vi "R45_2-RT.vi"() -> ()   [LabVIEW 2016]
uses:
  <vilib>/rvi/interface/nirviOpenFPGA/nirviOpenFPGA.xnode
  <vilib>/rvi/interface/nirviReadWriteControl/nirviReadWriteControl.xnode
  R45_2-FPGA.vi
  Controls/GP307 cluster.ctl
  <vilib>/functionblocks/FB Core/FB Core.xnode
  <vilib>/functionblocks/Control/PID/PID.vi
  <vilib>/functionblocks/NI_FunctionBlock Libraries.lvlib
  Controls/Glassman Control.ctl
  NiFpgaLv.dll
  <vilib>/Utility/error.llb/Error Cluster From Error Code.vi
  <vilib>/rvi/errors/niLvFpgaAdjustHostInterfaceError.vi
  Controls/GV states.ctl
  Controls/Aperture states.ctl
  Controls/Faraday cup states.ctl
  <vilib>/NI_Real-Time Target Support.lvlib
  FPGA Bitfiles/PRIMEControl2017_FPGATarget8_R45-2-FPGA_U4jwOoavuXQ.lvbitx
  <vilib>/FPGAPlugInAG/cRIO-9074/niLvFpga_Open_cRIO-9074.vi
panel:
  in  "Tab Control":T1(tab)
  out "R45 ExB 1 HV Enable":bool
  out "R45 ExB 1 voltage set":dbl
  out "ExB 1- I read":dbl
  out "ExB 1- V read":dbl
  out "ExB 2+ I read":dbl
  out "ExB 2+ V read":dbl
  out "ExB 2- I read":dbl
  out "ExB 2- V read":dbl
  out "R45 ExB 2 HV Enable":bool
  out "R45 ExB 2 voltage set":dbl
  out "X-Steerer Magnet current set":dbl
  out "ExB 1+ I read":dbl
  out "ExB 1+ V read":dbl
  out "GRM magnet current set":dbl
  out "GFM read string":string
  in  "proportional gain (Kc) - GFM":dbl=1.0
  in  "integral time (Ti, min) - GFM":dbl=0.01
  in  "derivative time (Td, min) - GFM":dbl
  in  "output high - GFM":dbl=205.0
  in  "output low - GFM":dbl
  out "GFM field read":u8[](array[numeric])
  out "GFM field":dbl format="%#_8f"
  out "GFM command":u8[](array[numeric])
  out "R45 ExB 2 command string":string
  out "R45 ExB 2 command array":u8[](array[numeric])
  out "ExB #2 magnet current set":dbl
  out "GFM command string":string
  out "GFM field set":dbl
  out "ExB #1 magnet current set":dbl
  out "R45 ExB 1 command string":string
  out "R45 ExB 1 command array":u8[](array[numeric])
  out "X-steerer Mag V read":dbl
  out "X-steerer Mag I read":dbl
  out "Ion Gauge 3-2":u8[](array[numeric])
  out "Convectron gauge 3-2":u8[](array[numeric])
  out "Ion gauge 2-2":u8[](array[numeric])
  out "Ion gauge 2-1":u8[](array[numeric])
  out "Convectron 3-1":u8[](array[numeric])
  out "Ion gauge 3-1":u8[](array[numeric])
  out "Convectron 2-2":u8[](array[numeric])
  out "Convectron 2-1":u8[](array[numeric])
  out "Ion Gauge 4-1":u8[](array[numeric])
  out "Convectron Gauge 4-1":u8[](array[numeric])
  out "Ion Gauge 4-2":u8[](array[numeric])
  out "Convectron Gauge 4-2":u8[](array[numeric])
  out "R45 Quad  vac gauge cluster":T2
  out "R45 Detector vac gauge cluster":T2
  out "R45 ExB Slot vac gauge cluster":T2
  out "Vac cluster 2 Ion Guage Interlock":bool
  out "Vac cluster 3 Ion Guage Interlock":bool
  out "Vac cluster 4 Ion Guage Interlock":bool
  out "Vac cluster 1 Gauge Interlock":bool
  out "Vac cluster 1 Interlock bypass":bool
  out "Switch Object Vac Interlock":bool
  out "Switch Object Interlock Bypass":bool
  out "Vac cluster 2 Interlock bypass":bool
  out "Vac cluster 4 Interlock bypass":bool
  out "Vac cluster 3 Interlock bypass":bool
  out "Turbo 2 GV Status":T3
  out "Turbo 1 GV Status":T3
  out "Beamline GV 3 Status":T3
  out "Beamline GV 2 Status":T3
  out "R45 Switching Mag GV Status":T3
  out "Turbo 3 GV Status":T3
  out "Detector FC status":T4
  out "Detector Aperture status":T5
  out "Detector Aperture Position":cluster{"IN sensor":bool, "OUT sensor":bool}
  out "Turbo 3 GV Status":T6
  out "Turbo 2 GV Status":T6
  out "Beamline GV 3 Status":T6
  out "Turbo 1 GV Status":T6
  out "R45 Switching Mag GV Status":T6
  out "ExB Slot Aperture Position":cluster{"IN sensor":bool, "OUT sensor":bool}
  out "Detector FC Position":cluster{"IN sensor":bool, "OUT sensor":bool}
  out "Beamline GV 2 Status":T6
  out "ExB Slot Aperture Status":T5
  out "R45 Detector FC insert":bool
  out "R45 Detector Aperture insert":bool
  out "R45 ExB Slot Aperture insert":bool
  out "R45 Turbo 3 GV":bool
  out "R45 Turbo 2 GV":bool
  out "R45 Switching Magnet GV":bool
  out "R45 Turbo 1 GV":bool
  out "R45 Beamline GV 3":bool
  out "R45 Beamline GV 2":bool
  out "HV control loop error":errorcluster
  out "HV readback loop error":errorcluster
  out "Error Reporter":errorcluster
  out "ExB 1 PS loop error":errorcluster
  out "ExB 2 PS loop error":errorcluster
  out "GFM loop error":errorcluster
  out "Interlock readbacks Loop error":errorcluster
  out "Vacuum readback error":errorcluster
  out "Actuator loop error":errorcluster
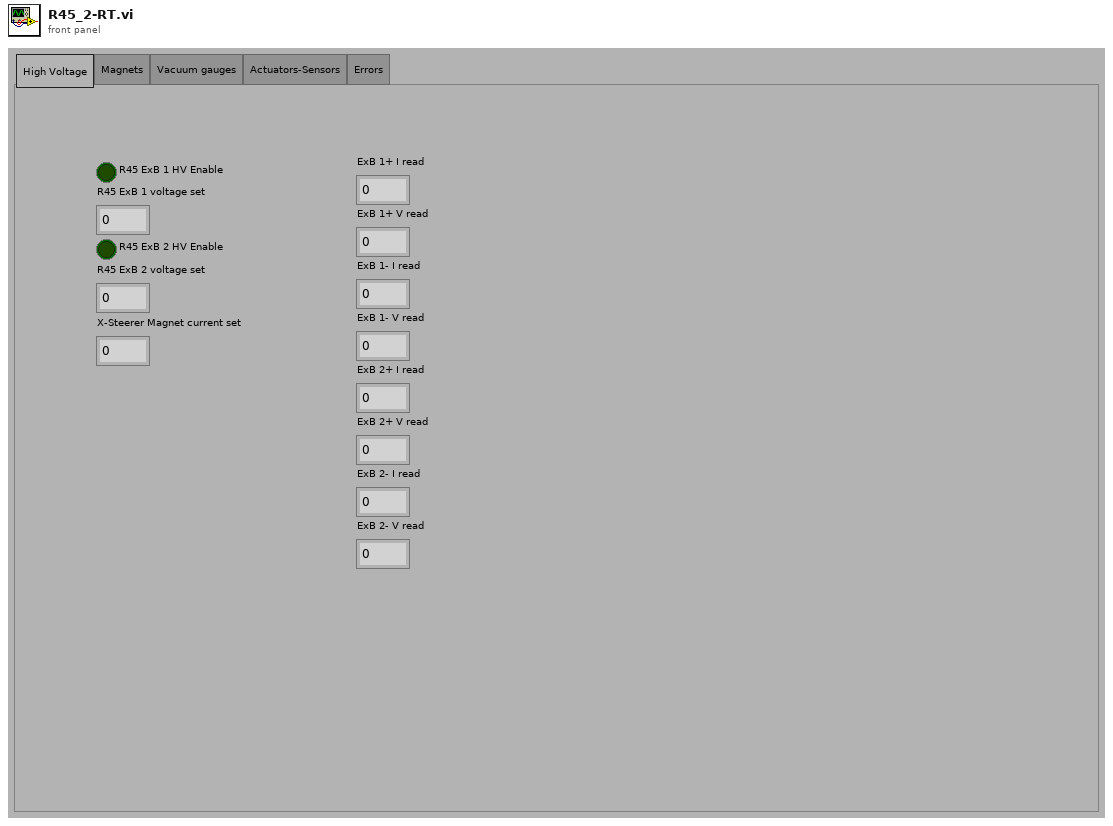
[diagram p1: front panel]
types:
  T1 = enum32{"High Voltage", "Magnets", "Vacuum gauges", "Actuators-Sensors", "Errors"}
  T2 = cluster{"Ion gauge 1":string, "Convectron  Gauge 1 ":string, "Ion Gauge 2":string, "Convectrom Gauge 2":string}
  T3 = typedef "GV states.ctl" = enum16{"status unclear", "closed", "open"}
  T4 = typedef "Faraday cup states.ctl" = enum16{"FC status unclear", "FC in", "FC out"}
  T5 = typedef "Aperture states.ctl" = enum16{"Aperture status unclear", "Aperture in", "Aperture out"}
  T6 = cluster{"OPEN sensor":bool, "Closed sensor":bool}
  T7 = typedef "Glassman Control.ctl" = cluster{"V-program":fxp<+/-,16,5>, "HV Enable":bool}
  T8 = cluster{"I-monitor":fxp<+/-,16,5>, "V-monitor":fxp<+/-,16,5>}
  T9 = typedef "GP307 cluster.ctl" = cluster{"Ion gauge 1":string, "Convectron  Gauge 1 ":string, "Ion Gauge 2":string, "Convectrom Gauge 2":string}
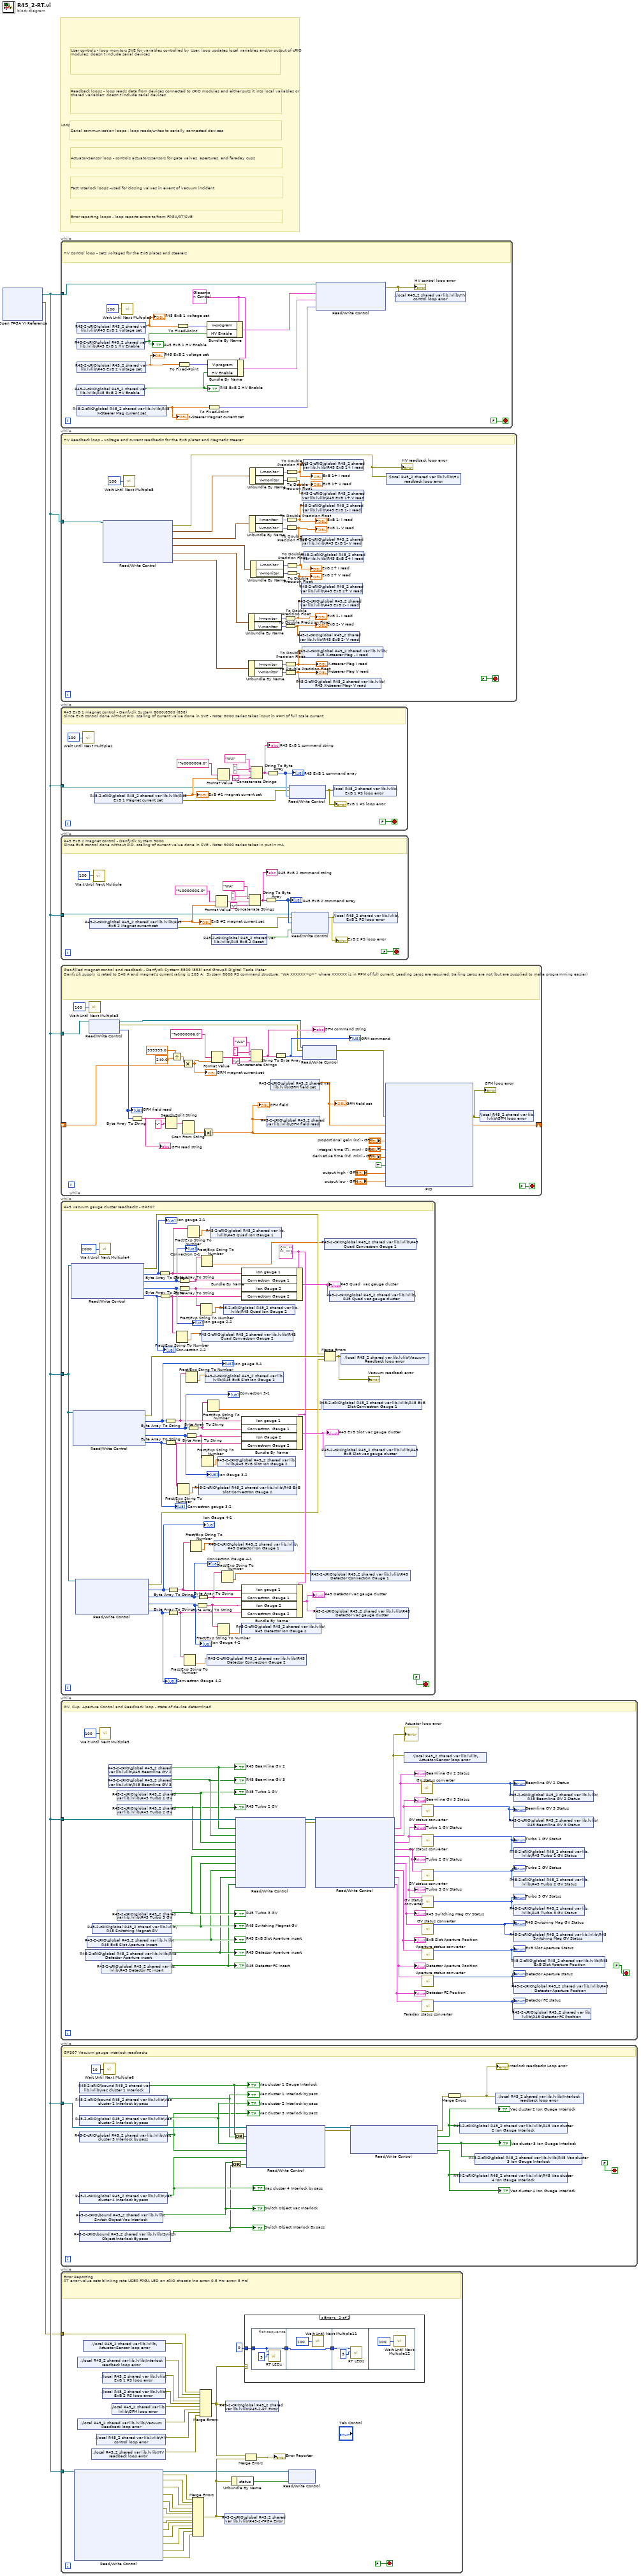
[diagram p0: block diagram]
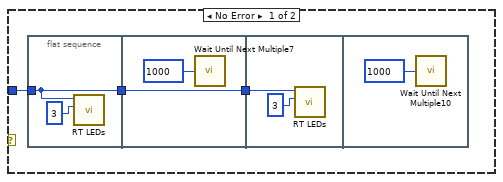
[diagram p2: hidden frame]
diagram:
  # "Serial communication loops - loop reads/writes to serially connected devices"
  # "Actuator-Sensor loop - controls actuators/sensors for gate valves, apertures, and faraday cups"
  # "Fast Interlock loops -used for closing valves in event of vacuum incident"
  # "Error reporting loops - loop reports errors to/from FPGA/RT/SVE"
  # "Readback loops - loop reads data from devices connected to cRIO modules and either puts it into local variables or shared variables; doesn't include serial devices"
  # "User controls - loop monitors SVE for variables controlled by User; loop updates local variables and/or output of cRIO modules; doesn't include serial devices"
  # "Loop legend - loops are color coded by responsibility"
  n1 = xnode "Open FPGA VI Reference"() -> ("FPGA VI Reference Out"=w2:refnum<k20>, "error out"=w1:errorcluster)  [unwired: 2 in]
  n2 = while {
    tunnel: w2 -> [w17]
    stop <- FALSE stop-if-true
    w13 = T7 {"V-program"=0.0, "HV Enable"=FALSE} ("Glassman Control")
    # "HV Control loop - sets voltages for the ExB plates and steerers"
    n3 = shared-variable "R45-2-cRIO\\global R45_2 shared var lib.lvlib\\R45 ExB 1 voltage set"() -> (w10:dbl)  [unwired: 1 in, 1 out]
    "R45 ExB 1 voltage set" <- w10
    n4 = shared-variable "R45-2-cRIO\\global R45_2 shared var lib.lvlib\\R45 ExB 1 HV Enable"() -> (w11:bool)  [unwired: 1 in, 1 out]
    "R45 ExB 1 HV Enable" <- w11
    n5 = shared-variable "R45-2-cRIO\\global R45_2 shared var lib.lvlib\\R45 ExB 2 voltage set"() -> (w8:dbl)  [unwired: 1 in, 1 out]
    "R45 ExB 2 voltage set" <- w8
    n6 = shared-variable "R45-2-cRIO\\global R45_2 shared var lib.lvlib\\R45 ExB 2 HV Enable"() -> (w6:bool)  [unwired: 1 in, 1 out]
    "R45 ExB 2 HV Enable" <- w6
    n7 = shared-variable "R45-2-cRIO\\global R45_2 shared var lib.lvlib\\R45 X-Steerer Mag current set"() -> (w16:dbl)  [unwired: 1 in, 1 out]
    "X-Steerer Magnet current set" <- w16
    n8 = call "Wait Until Next Multiple9"("Count(mSec)"=u32 100 ("millisecond multiple")) -> ()  [unwired: 1 out]
    n9 = To Fixed-Point(number=w10) -> (fixed-point=w9:fxp<+/-,20,5>)  [unwired: 1 in]
    n10 = To Fixed-Point(number=w8) -> (fixed-point=w7:fxp<+/-,20,5>)  [unwired: 1 in]
    n11 = Bundle By Name(cluster=w13, "V-program"=w9, "HV Enable"=w11) -> (w12:T7)
    n12 = Bundle By Name(cluster=w13, "V-program"=w7, "HV Enable"=w6) -> (w14:T7)
    n13 = To Fixed-Point(number=w16) -> (fixed-point=w15:fxp<+/-,20,5>)  [unwired: 1 in]
    n14 = xnode "Read/Write Control"("FPGA VI Reference In"=w17, "ExB 1 - Voltage Set"=w12, "ExB 2 - Voltage Set"=w14, "Mag Steerer I-program"=w15) -> ("error out"=w5:errorcluster)  [unwired: 1 in, 1 out]
    "HV control loop error" <- w5
    n15 = shared-variable ".\\local R45_2 shared var lib.lvlib\\HV control loop error"(w5) -> ()  [unwired: 1 in, 1 out]
  }
  n16 = while {
    tunnel: w2 -> [w46]
    stop <- FALSE stop-if-true
    # "HV Readback loop - voltage and current readbacks for the ExB plates and Magnetic steerer"
    n17 = xnode "Read/Write Control"("FPGA VI Reference In"=w46) -> ("error out"=w28:errorcluster, "ExB 1+ Monitor"=w45:T8, "ExB 1- Monitor"=w44:T8, "ExB 2+ Monitor"=w43:T8, "ExB 2- Monitor"=w42:T8, "Mag Steerer - Monitor"=w41:T8)  [unwired: 1 in, 1 out]
    "HV readback loop error" <- w28
    n18 = call "Wait Until Next Multiple8"("Count(mSec)"=u32 100 ("millisecond multiple")) -> ()  [unwired: 1 out]
    n19 = Unbundle By Name(w42) -> ("I-monitor"=w35:fxp<+/-,16,5>, "V-monitor"=w34:fxp<+/-,16,5>)
    n20 = Unbundle By Name(w41) -> ("I-monitor"=w33:fxp<+/-,16,5>, "V-monitor"=w32:fxp<+/-,16,5>)
    n21 = Unbundle By Name(w44) -> ("I-monitor"=w39:fxp<+/-,16,5>, "V-monitor"=w38:fxp<+/-,16,5>)
    n22 = Unbundle By Name(w45) -> ("I-monitor"=w31:fxp<+/-,16,5>, "V-monitor"=w40:fxp<+/-,16,5>)
    n23 = Unbundle By Name(w43) -> ("I-monitor"=w37:fxp<+/-,16,5>, "V-monitor"=w36:fxp<+/-,16,5>)
    n24 = To Double Precision Float(number=w35) -> (double precision float=w22:dbl)
    "ExB 2- I read" <- w22
    n25 = To Double Precision Float(number=w34) -> (double precision float=w21:dbl)
    "ExB 2- V read" <- w21
    n26 = To Double Precision Float(number=w33) -> (double precision float=w20:dbl)
    "X-steerer Mag I read" <- w20
    n27 = To Double Precision Float(number=w32) -> (double precision float=w19:dbl)
    "X-steerer Mag V read" <- w19
    n28 = To Double Precision Float(number=w39) -> (double precision float=w26:dbl)
    "ExB 1- I read" <- w26
    n29 = To Double Precision Float(number=w38) -> (double precision float=w25:dbl)
    "ExB 1- V read" <- w25
    n30 = To Double Precision Float(number=w31) -> (double precision float=w29:dbl)
    "ExB 1+ I read" <- w29
    n31 = To Double Precision Float(number=w40) -> (double precision float=w30:dbl)
    "ExB 1+ V read" <- w30
    n32 = To Double Precision Float(number=w37) -> (double precision float=w24:dbl)
    "ExB 2+ I read" <- w24
    n33 = To Double Precision Float(number=w36) -> (double precision float=w23:dbl)
    "ExB 2+ V read" <- w23
    n34 = shared-variable "R45-2-cRIO\\global R45_2 shared var lib.lvlib\\R45 ExB 2- V read"(w21) -> ()  [unwired: 1 in, 1 out]
    n35 = shared-variable "R45-2-cRIO\\global R45_2 shared var lib.lvlib\\R45 X-steerer Mag- V read"(w19) -> ()  [unwired: 1 in, 1 out]
    n36 = shared-variable "R45-2-cRIO\\global R45_2 shared var lib.lvlib\\R45 ExB 2+ V read"(w23) -> ()  [unwired: 1 in, 1 out]
    n37 = shared-variable "R45-2-cRIO\\global R45_2 shared var lib.lvlib\\R45 ExB 2- I read"(w22) -> ()  [unwired: 1 in, 1 out]
    n38 = shared-variable "R45-2-cRIO\\global R45_2 shared var lib.lvlib\\R45 ExB 1- V read"(w25) -> ()  [unwired: 1 in, 1 out]
    n39 = shared-variable "R45-2-cRIO\\global R45_2 shared var lib.lvlib\\R45 X-steerer Mag - I read"(w20) -> ()  [unwired: 1 in, 1 out]
    n40 = shared-variable "R45-2-cRIO\\global R45_2 shared var lib.lvlib\\R45 ExB 1+ V read"(w30) -> ()  [unwired: 1 in, 1 out]
    n41 = shared-variable "R45-2-cRIO\\global R45_2 shared var lib.lvlib\\R45 ExB 1- I read"(w26) -> ()  [unwired: 1 in, 1 out]
    n42 = shared-variable "R45-2-cRIO\\global R45_2 shared var lib.lvlib\\R45 ExB 1+ I read"(w29) -> ()  [unwired: 1 in, 1 out]
    n43 = shared-variable "R45-2-cRIO\\global R45_2 shared var lib.lvlib\\R45 ExB 2+ I read"(w24) -> ()  [unwired: 1 in, 1 out]
    n44 = shared-variable ".\\local R45_2 shared var lib.lvlib\\HV readback loop error"(w28) -> ()  [unwired: 1 in, 1 out]
  }
  n45 = while {
    tunnel: w2 -> [w50]
    stop <- FALSE stop-if-true
    # "R45 ExB 1 magnet control - Danfysik System 8000/8500 (858)\nSince ExB control done without PID, scaling of current value done in SVE - Note: 8000 series takes input in PPM of full scale current"
    n46 = call "Wait Until Next Multiple2"("Count(mSec)"=u32 100 ("millisecond multiple")) -> ()  [unwired: 1 out]
    n47 = shared-variable "R45-2-cRIO\\global R45_2 shared var lib.lvlib\\R45 ExB 1 Magnet current set"() -> (w57:dbl, error out=w51:errorcluster)  [unwired: 1 in]
    "ExB #1 magnet current set" <- w57
    n48 = Format Value(format string="%0000006.0", value (0)=w57) -> (output string=w55:string)  [unwired: 1 out]
    n49 = Concatenate Strings("WA", " ", w55, "\r") -> (w58:string)
    "R45 ExB 1 command string" <- w58
    n50 = String To Byte Array(string=w58) -> (unsigned byte array=w56:u8[])
    "R45 ExB 1 command array" <- w56
    n51 = xnode "Read/Write Control"("FPGA VI Reference In"=w50, "error in"=w51, "ExB 1 PS set"=w56) -> ("error out"=w48:errorcluster)  [unwired: 1 out]
    "ExB 1 PS loop error" <- w48
    n52 = shared-variable ".\\local R45_2 shared var lib.lvlib\\ExB 1 PS loop error"(w48) -> ()  [unwired: 1 in, 1 out]
  }
  n53 = while {
    tunnel: w2 -> [w62]
    stop <- FALSE stop-if-true
    # "R45 ExB 2 magnet control - Danfysik System 9000\nSince ExB control done without PID, scaling of current value done in SVE - Note: 9000 series takes in put in mA"
    n54 = shared-variable "R45-2-cRIO\\global R45_2 shared var lib.lvlib\\R45 ExB 2 Magnet current set"() -> (w70:dbl, error out=w64:errorcluster)  [unwired: 1 in]
    "ExB #2 magnet current set" <- w70
    n55 = call "Wait Until Next Multiple"("Count(mSec)"=u32 100 ("millisecond multiple")) -> ()  [unwired: 1 out]
    n56 = shared-variable "R45-2-cRIO\\global R45_2 shared var lib.lvlib\\R45 ExB 2 Reset"() -> (w73:bool)  [unwired: 1 in, 1 out]
    n57 = Format Value(format string="%0000006.0", value (0)=w70) -> (output string=w68:string)  [unwired: 1 out]
    n58 = Concatenate Strings("WA", " ", w68, "\r") -> (w71:string)
    "R45 ExB 2 command string" <- w71
    n59 = String To Byte Array(string=w71) -> (unsigned byte array=w69:u8[])
    "R45 ExB 2 command array" <- w69
    n60 = xnode "Read/Write Control"("FPGA VI Reference In"=w62, "error in"=w64, "ExB 2 PS set"=w69, "ExB 2 Reset"=w73) -> ("error out"=w63:errorcluster)  [unwired: 1 out]
    "ExB 2 PS loop error" <- w63
    n61 = shared-variable ".\\local R45_2 shared var lib.lvlib\\ExB 2 PS loop error"(w63) -> ()  [unwired: 1 in, 1 out]
  }
  n62 = while {
    tunnel: w2 -> [w97]
    shift-right: [w92] -> _
    shift-left: _ -> [w86]
    stop <- FALSE stop-if-true
    # "Gas-filled magnet control and readback - Danfysik System 8500 (853) and Group3 Digital Tesla Meter\nDanfysik supply is rated to 240 A and magnet's current rating is 205 A;  System 8000 PS command structure: \"WA XXXXXX<cr>\" where XXXXXX is in PPM of full current. Leading zeros are required; trailing zeros are not (but are supplied to make programming easier)"
    n63 = call "Wait Until Next Multiple3"("Count(mSec)"=u32 100 ("millisecond multiple")) -> ()  [unwired: 1 out]
    n64 = xnode "Read/Write Control"("FPGA VI Reference In"=w97) -> ("FPGA VI Reference Out"=w96:refnum<k20>, "error out"=w95:errorcluster, "GFM read"=w98:u8[])  [unwired: 1 in]
    "GFM field read" <- w98
    n65 = Byte Array To String(unsigned byte array=w98) -> (string=w76:string)
    "GFM read string" <- w76
    n66 = Search/Split String(string=w76, search string/char (-)="-") -> (match + rest of string=w77:string)  [unwired: 3 out]
    n67 = Divide(x=999999.0, y=240.0) -> (x/y=w82:dbl)
    n68 = Multiply(x=w82, y=w86) -> (x*y=w83:dbl)
    "GRM magnet current set" <- w83
    n69 = Scan From String(input string=w77) -> (output 1=w78:dbl)  [unwired: 3 in, 4 out]
    n70 = Absolute Value(x=w78) -> (abs(x)=w75:dbl)
    "GFM field" <- w75
    n71 = Format Value(format string="%0000006.0", value (0)=w83) -> (output string=w104:string)  [unwired: 1 out]
    n72 = Concatenate Strings("WA", " ", w104, "\r") -> (w100:string)
    "GFM command string" <- w100
    n73 = shared-variable "R45-2-cRIO\\global R45_2 shared var lib.lvlib\\GFM field read"(w75) -> ()  [unwired: 1 in, 1 out]
    n74 = shared-variable "R45-2-cRIO\\global R45_2 shared var lib.lvlib\\GFM field set"() -> (w91:dbl)  [unwired: 1 in, 1 out]
    "GFM field set" <- w91
    n75 = String To Byte Array(string=w100) -> (unsigned byte array=w99:u8[])
    "GFM command" <- w99
    n76 = xnode "Read/Write Control"("FPGA VI Reference In"=w96, "error in"=w95, "GFM ps set"=w99) -> ("error out"=w94:errorcluster)  [unwired: 1 out]
    n77 = xnode "PID"("error in"=w94, "setpoint"=w91, "process variable"=w75, "proportional gain (Kc)"="proportional gain (Kc) - GFM", "integral time (Ti, min)"="integral time (Ti, min) - GFM", "derivative time (Td, min)"="derivative time (Td, min) - GFM", "auto? (T)"=TRUE, "output high"="output high - GFM", "output low"="output low - GFM") -> ("error out"=w93:errorcluster, "output"=w92:dbl)
    "GFM loop error" <- w93
    n78 = shared-variable ".\\local R45_2 shared var lib.lvlib\\GFM loop error"(w93) -> ()  [unwired: 1 in, 1 out]
  }
  n79 = while {
    tunnel: w2 -> [w197]
    stop <- FALSE stop-if-true
    w208 = T9 {"Ion gauge 1"="", "Convectron  Gauge 1 "="", "Ion Gauge 2"="", "Convectrom Gauge 2"=""} ("Ion gauge cluster control")
    # "R45 vacuum gauge cluster readbacks - GP307"
    n80 = xnode "Read/Write Control"("FPGA VI Reference In"=w197) -> ("error out"=w187:errorcluster, "Vac Cluster 2 Ion Gauge 1"=w196:u8[], "Vac Cluster 2 Convectron 1"=w195:u8[], "Vac Cluster 2 Ion Gauge 2"=w194:u8[], "Vac Cluster 2 Convectron 2"=w193:u8[])  [unwired: 1 in, 1 out]
    "Ion gauge 2-1" <- w196
    "Convectron 2-1" <- w195
    "Ion gauge 2-2" <- w194
    "Convectron 2-2" <- w193
    n81 = xnode "Read/Write Control"("FPGA VI Reference In"=w197) -> ("error out"=w219:errorcluster, "Vac Cluster 3 Ion Gauge 1"=w217:u8[], "Vac Cluster 3 Convectron 1"=w216:u8[], "Vac Cluster 3 Ion Gauge 2"=w214:u8[], "Vac Cluster 3 Convectron 2"=w215:u8[])  [unwired: 1 in, 1 out]
    "Ion gauge 3-1" <- w217
    "Convectron 3-1" <- w216
    "Convectron gauge 3-2" <- w215
    "Ion Gauge 3-2" <- w214
    n82 = xnode "Read/Write Control"("FPGA VI Reference In"=w197) -> ("error out"=w186:errorcluster, "Vac Cluster 4 Ion Gauge 1"=w200:u8[], "Vac Cluster 4 Convectron 1"=w202:u8[], "Vac Cluster 4 Ion Gauge 2"=w203:u8[], "Vac Cluster 4 Convectron 2"=w201:u8[])  [unwired: 1 in, 1 out]
    "Ion Gauge 4-1" <- w200
    "Convectron Gauge 4-1" <- w202
    "Ion Gauge 4-2" <- w203
    "Convectron Gauge 4-2" <- w201
    n83 = call "Wait Until Next Multiple4"("Count(mSec)"=u32 2000 ("millisecond multiple")) -> ()  [unwired: 1 out]
    n84 = Byte Array To String(unsigned byte array=w196) -> (string=w212:string)
    n85 = Byte Array To String(unsigned byte array=w193) -> (string=w190:string)
    n86 = Byte Array To String(unsigned byte array=w217) -> (string=w211:string)
    n87 = Byte Array To String(unsigned byte array=w215) -> (string=w192:string)
    n88 = Byte Array To String(unsigned byte array=w200) -> (string=w204:string)
    n89 = Byte Array To String(unsigned byte array=w201) -> (string=w198:string)
    n90 = Fract/Exp String To Number(string=w190) -> (number=w175:dbl)  [unwired: 3 in, 1 out]
    n91 = Fract/Exp String To Number(string=w192) -> (number=w179:dbl)  [unwired: 3 in, 1 out]
    n92 = Byte Array To String(unsigned byte array=w195) -> (string=w209:string)
    n93 = Byte Array To String(unsigned byte array=w194) -> (string=w189:string)
    n94 = Fract/Exp String To Number(string=w198) -> (number=w182:dbl)  [unwired: 3 in, 1 out]
    n95 = Fract/Exp String To Number(string=w211) -> (number=w181:dbl)  [unwired: 3 in, 1 out]
    n96 = Byte Array To String(unsigned byte array=w214) -> (string=w191:string)
    n97 = Fract/Exp String To Number(string=w212) -> (number=w177:dbl)  [unwired: 3 in, 1 out]
    n98 = Byte Array To String(unsigned byte array=w216) -> (string=w210:string)
    n99 = Fract/Exp String To Number(string=w204) -> (number=w185:dbl)  [unwired: 3 in, 1 out]
    n100 = Byte Array To String(unsigned byte array=w203) -> (string=w199:string)
    n101 = Byte Array To String(unsigned byte array=w202) -> (string=w205:string)
    n102 = shared-variable "R45-2-cRIO\\global R45_2 shared var lib.lvlib\\R45 ExB Slot Convectron Gauge 2"(w179) -> ()  [unwired: 1 in, 1 out]
    n103 = Fract/Exp String To Number(string=w189) -> (number=w176:dbl)  [unwired: 3 in, 1 out]
    n104 = Fract/Exp String To Number(string=w209) -> (number=w174:dbl)  [unwired: 3 in, 1 out]
    n105 = shared-variable "R45-2-cRIO\\global R45_2 shared var lib.lvlib\\R45 Quad Convectron Gauge 2"(w175) -> ()  [unwired: 1 in, 1 out]
    n106 = Fract/Exp String To Number(string=w191) -> (number=w180:dbl)  [unwired: 3 in, 1 out]
    n107 = shared-variable "R45-2-cRIO\\global R45_2 shared var lib.lvlib\\R45 ExB Slot Ion Gauge 1"(w181) -> ()  [unwired: 1 in, 1 out]
    n108 = shared-variable "R45-2-cRIO\\global R45_2 shared var lib.lvlib\\R45 Detector Convectron Gauge 2"(w182) -> ()  [unwired: 1 in, 1 out]
    n109 = Fract/Exp String To Number(string=w210) -> (number=w178:dbl)  [unwired: 3 in, 1 out]
    n110 = shared-variable "R45-2-cRIO\\global R45_2 shared var lib.lvlib\\R45 Quad Ion Gauge 1"(w177) -> ()  [unwired: 1 in, 1 out]
    n111 = shared-variable "R45-2-cRIO\\global R45_2 shared var lib.lvlib\\R45 Detector Ion Gauge 1"(w185) -> ()  [unwired: 1 in, 1 out]
    n112 = shared-variable "R45-2-cRIO\\global R45_2 shared var lib.lvlib\\R45 ExB Slot Ion Gauge 2"(w180) -> ()  [unwired: 1 in, 1 out]
    n113 = Fract/Exp String To Number(string=w199) -> (number=w184:dbl)  [unwired: 3 in, 1 out]
    n114 = Fract/Exp String To Number(string=w205) -> (number=w183:dbl)  [unwired: 3 in, 1 out]
    n115 = shared-variable "R45-2-cRIO\\global R45_2 shared var lib.lvlib\\R45 Quad Ion Gauge 2"(w176) -> ()  [unwired: 1 in, 1 out]
    n116 = shared-variable "R45-2-cRIO\\global R45_2 shared var lib.lvlib\\R45 Detector Ion Gauge 2"(w184) -> ()  [unwired: 1 in, 1 out]
    n117 = Bundle By Name(cluster=w208, "Ion gauge 1"=w212, "Convectron  Gauge 1"=w209, "Ion Gauge 2"=w189, "Convectrom Gauge 2"=w190) -> (w213:T9)
    "R45 Quad  vac gauge cluster" <- w213
    n118 = Bundle By Name(cluster=w208, "Ion gauge 1"=w211, "Convectron  Gauge 1"=w210, "Ion Gauge 2"=w192, "Convectrom Gauge 2"=w191) -> (w206:T9)
    "R45 ExB Slot vac gauge cluster" <- w206
    n119 = Bundle By Name(cluster=w208, "Ion gauge 1"=w204, "Convectron  Gauge 1"=w205, "Ion Gauge 2"=w199, "Convectrom Gauge 2"=w198) -> (w207:T9)
    "R45 Detector vac gauge cluster" <- w207
    n120 = shared-variable "R45-2-cRIO\\global R45_2 shared var lib.lvlib\\R45 Detector Convectron Gauge 1"(w183) -> ()  [unwired: 1 in, 1 out]
    n121 = shared-variable "R45-2-cRIO\\global R45_2 shared var lib.lvlib\\R45 Detector vac gauge cluster"(w207) -> ()  [unwired: 1 in, 1 out]
    n122 = shared-variable "R45-2-cRIO\\global R45_2 shared var lib.lvlib\\R45 ExB Slot Convectron Gauge 1"(w178) -> ()  [unwired: 1 in, 1 out]
    n123 = shared-variable "R45-2-cRIO\\global R45_2 shared var lib.lvlib\\R45 Quad Convectron Gauge 1"(w174) -> ()  [unwired: 1 in, 1 out]
    n124 = Merge Errors(w187, w219, w186) -> (w188:errorcluster)
    "Vacuum readback error" <- w188
    n125 = shared-variable "R45-2-cRIO\\global R45_2 shared var lib.lvlib\\R45 ExB Slot vac gauge cluster"(w206) -> ()  [unwired: 1 in, 1 out]
    n126 = shared-variable "R45-2-cRIO\\global R45_2 shared var lib.lvlib\\R45 Quad vac gauge cluster"(w213) -> ()  [unwired: 1 in, 1 out]
    n127 = shared-variable ".\\local R45_2 shared var lib.lvlib\\Vacuum Readback loop error"(w188) -> ()  [unwired: 1 in, 1 out]
  }
  n128 = while {
    tunnel: w2 -> [w251]
    stop <- FALSE stop-if-true
    # "GV, Cup, Aperture Control and Readback loop - state of device determined"
    n129 = shared-variable "R45-2-cRIO\\global R45_2 shared var lib.lvlib\\R45 Detector Aperture insert"() -> (w241:bool)  [unwired: 1 in, 1 out]
    "R45 Detector Aperture insert" <- w241
    n130 = shared-variable "R45-2-cRIO\\global R45_2 shared var lib.lvlib\\R45 ExB Slot Aperture insert"() -> (w242:bool)  [unwired: 1 in, 1 out]
    "R45 ExB Slot Aperture insert" <- w242
    n131 = shared-variable "R45-2-cRIO\\global R45_2 shared var lib.lvlib\\R45 Switching Magnet GV"() -> (w243:bool)  [unwired: 1 in, 1 out]
    "R45 Switching Magnet GV" <- w243
    n132 = call "Wait Until Next Multiple5"("Count(mSec)"=u32 100 ("millisecond multiple")) -> ()  [unwired: 1 out]
    n133 = shared-variable "R45-2-cRIO\\global R45_2 shared var lib.lvlib\\R45 Detector FC insert"() -> (w240:bool)  [unwired: 1 in, 1 out]
    "R45 Detector FC insert" <- w240
    n134 = shared-variable "R45-2-cRIO\\global R45_2 shared var lib.lvlib\\R45 Beamline GV 2"() -> (w248:bool)  [unwired: 1 in, 1 out]
    "R45 Beamline GV 2" <- w248
    n135 = shared-variable "R45-2-cRIO\\global R45_2 shared var lib.lvlib\\R45 Beamline GV 3"() -> (w247:bool)  [unwired: 1 in, 1 out]
    "R45 Beamline GV 3" <- w247
    n136 = shared-variable "R45-2-cRIO\\global R45_2 shared var lib.lvlib\\R45 Turbo 1 GV"() -> (w246:bool)  [unwired: 1 in, 1 out]
    "R45 Turbo 1 GV" <- w246
    n137 = shared-variable "R45-2-cRIO\\global R45_2 shared var lib.lvlib\\R45 Turbo 2 GV"() -> (w245:bool)  [unwired: 1 in, 1 out]
    "R45 Turbo 2 GV" <- w245
    n138 = shared-variable "R45-2-cRIO\\global R45_2 shared var lib.lvlib\\R45 Turbo 3 GV"() -> (w244:bool)  [unwired: 1 in, 1 out]
    "R45 Turbo 3 GV" <- w244
    n139 = xnode "Read/Write Control"("FPGA VI Reference In"=w251, "Beamline GV 2"=w248, "Beamline GV 3"=w247, "Turbo 1 GV"=w246, "Turbo 2 GV"=w245, "Turbo 3 GV"=w244, "Switching Magnet GV"=w243, "ExB Slot Aperture insert"=w242, "Detector Aperture insert"=w241, "Detector FC insert"=w240) -> ("FPGA VI Reference Out"=w250:refnum<k20>, "error out"=w249:errorcluster)  [unwired: 1 in]
    n140 = xnode "Read/Write Control"("FPGA VI Reference In"=w250, "error in"=w249) -> ("error out"=w239:errorcluster, "Beamline GV 2 Status"=w227:T6, "Beamline GV 3 Status"=w228:T6, "Turbo 1 GV Status"=w226:T6, "Turbo 2 GV Status"=w229:T6, "Turbo 3 GV Status"=w230:T6, "R45 Switching Mag GV Status"=w232:T6, "ExB Slot Aperture Position"=w234:cluster{"IN sensor":bool, "OUT sensor":bool}, "Detector Aperture Position"=w236:cluster{"IN sensor":bool, "OUT sensor":bool}, "Detector FC Position"=w238:cluster{"IN sensor":bool, "OUT sensor":bool})  [unwired: 1 out]
    "Beamline GV 2 Status" <- w227
    "Beamline GV 3 Status" <- w228
    "Turbo 1 GV Status" <- w226
    "Turbo 2 GV Status" <- w229
    "Turbo 3 GV Status" <- w230
    "R45 Switching Mag GV Status" <- w232
    "ExB Slot Aperture Position" <- w234
    "Detector Aperture Position" <- w236
    "Detector FC Position" <- w238
    "Actuator loop error" <- w239
    n141 = shared-variable ".\\local R45_2 shared var lib.lvlib\\Actuator-Sensor loop error"(w239) -> ()  [unwired: 1 in, 1 out]
    n142 = call "GV status converter.vi"("Gate Valve"=w227) -> ("GV Status"=w225:T3)  [unwired: 10 in]
    "Beamline GV 2 Status" <- w225
    n143 = call "GV status converter.vi"("Gate Valve"=w228) -> ("GV Status"=w224:T3)  [unwired: 10 in]
    "Beamline GV 3 Status" <- w224
    n144 = call "GV status converter.vi"("Gate Valve"=w226) -> ("GV Status"=w223:T3)  [unwired: 10 in]
    "Turbo 1 GV Status" <- w223
    n145 = call "GV status converter.vi"("Gate Valve"=w229) -> ("GV Status"=w222:T3)  [unwired: 10 in]
    "Turbo 2 GV Status" <- w222
    n146 = call "GV status converter.vi"("Gate Valve"=w230) -> ("GV Status"=w221:T3)  [unwired: 10 in]
    "Turbo 3 GV Status" <- w221
    n147 = call "GV status converter.vi"("Gate Valve"=w232) -> ("GV Status"=w231:T3)  [unwired: 10 in]
    "R45 Switching Mag GV Status" <- w231
    n148 = call "Aperture status converter.vi"("Aperture Position"=w234) -> ("Aperture Status"=w233:T5)  [unwired: 10 in]
    "ExB Slot Aperture Status" <- w233
    n149 = call "Aperture status converter.vi"("Aperture Position"=w236) -> ("Aperture Status"=w235:T5)  [unwired: 10 in]
    "Detector Aperture status" <- w235
    n150 = call "Faraday status converter.vi"("FC Position"=w238) -> ("FC Status"=w237:T4)  [unwired: 10 in]
    "Detector FC status" <- w237
    n151 = shared-variable "R45-2-cRIO\\global R45_2 shared var lib.lvlib\\R45 Beamline GV 2 Status"(w225) -> ()  [unwired: 1 in, 1 out]
    n152 = shared-variable "R45-2-cRIO\\global R45_2 shared var lib.lvlib\\R45 Beamline GV 3 Status"(w224) -> ()  [unwired: 1 in, 1 out]
    n153 = shared-variable "R45-2-cRIO\\global R45_2 shared var lib.lvlib\\R45 Turbo 1 GV Status"(w223) -> ()  [unwired: 1 in, 1 out]
    n154 = shared-variable "R45-2-cRIO\\global R45_2 shared var lib.lvlib\\R45 Turbo 2 GV Status"(w222) -> ()  [unwired: 1 in, 1 out]
    n155 = shared-variable "R45-2-cRIO\\global R45_2 shared var lib.lvlib\\R45 Turbo 3 GV Status"(w221) -> ()  [unwired: 1 in, 1 out]
    n156 = shared-variable "R45-2-cRIO\\global R45_2 shared var lib.lvlib\\R45 Switching Mag GV Status"(w231) -> ()  [unwired: 1 in, 1 out]
    n157 = shared-variable "R45-2-cRIO\\global R45_2 shared var lib.lvlib\\R45 ExB Slot Aperture Position"(w233) -> ()  [unwired: 1 in, 1 out]
    n158 = shared-variable "R45-2-cRIO\\global R45_2 shared var lib.lvlib\\R45 Detector Aperture Position"(w235) -> ()  [unwired: 1 in, 1 out]
    n159 = shared-variable "R45-2-cRIO\\global R45_2 shared var lib.lvlib\\R45 Detector FC Position"(w237) -> ()  [unwired: 1 in, 1 out]
  }
  n160 = while {
    tunnel: w2 -> [w259]
    stop <- FALSE stop-if-true
    # "GP307 Vacuum gauge interlock readbacks"
    n161 = shared-variable "R45-2-cRIO\\global R45_2 shared var lib.lvlib\\Vac cluster 3 Interlock bypass"() -> (w254:bool)  [unwired: 1 in, 1 out]
    "Vac cluster 3 Interlock bypass" <- w254
    n162 = shared-variable "R45-2-cRIO\\bound R45_2 shared var lib.lvlib\\Vac cluster 1 Interlock"() -> (w263:bool)  [unwired: 1 in, 1 out]
    "Vac cluster 1 Gauge Interlock" <- w263
    n163 = shared-variable "R45-2-cRIO\\bound R45_2 shared var lib.lvlib\\Vac cluster 1 Interlock bypass"() -> (w255:bool)  [unwired: 1 in, 1 out]
    "Vac cluster 1 Interlock bypass" <- w255
    n164 = shared-variable "R45-2-cRIO\\global R45_2 shared var lib.lvlib\\Vac cluster 2 Interlock bypass"() -> (w260:bool)  [unwired: 1 in, 1 out]
    "Vac cluster 2 Interlock bypass" <- w260
    n165 = shared-variable "R45-2-cRIO\\global R45_2 shared var lib.lvlib\\Vac cluster 4 Interlock bypass"() -> (w261:bool)  [unwired: 1 in, 1 out]
    "Vac cluster 4 Interlock bypass" <- w261
    n166 = shared-variable "R45-2-cRIO\\bound R45_2 shared var lib.lvlib\\Switch Object Vac Interlock"() -> (w262:bool)  [unwired: 1 in, 1 out]
    "Switch Object Vac Interlock" <- w262
    n167 = shared-variable "R45-2-cRIO\\bound R45_2 shared var lib.lvlib\\Switch Object Interlock Bypass"() -> (w257:bool)  [unwired: 1 in, 1 out]
    "Switch Object Interlock Bypass" <- w257
    n168 = call "Wait Until Next Multiple6"("Count(mSec)"=u32 10 ("millisecond multiple")) -> ()  [unwired: 1 out]
    n169 = Or(x=w262, y=w257) -> (x .or. y?=w258:bool)
    n170 = Or(x=w263, y=w255) -> (x .or. y?=w256:bool)
    n171 = xnode "Read/Write Control"("FPGA VI Reference In"=w259, "Vac cluster 1 Gauge Interlock"=w256, "Vac cluster 2 Interlock bypass"=w260, "Vac cluster 3 Interlock bypass"=w254, "Vac cluster 4 Interlock bypass"=w261, "Switch Object Interlock"=w258) -> ("FPGA VI Reference Out"=w265:refnum<k20>, "error out"=w264:errorcluster)  [unwired: 1 in]
    n172 = xnode "Read/Write Control"("FPGA VI Reference In"=w265, "error in"=w264) -> ("error out"=w267:errorcluster, "Vac cluster 2 Ion Gauge Interlock"=w268:bool, "Vac cluster 3 Ion Gauge Interlock"=w270:bool, "Vac cluster 4 Ion Gauge Interlock"=w269:bool)  [unwired: 1 out]
    "Vac cluster 2 Ion Guage Interlock" <- w268
    "Vac cluster 3 Ion Guage Interlock" <- w270
    "Vac cluster 4 Ion Guage Interlock" <- w269
    n173 = Merge Errors(w267) -> (w266:errorcluster)
    "Interlock readbacks Loop error" <- w266
    n174 = shared-variable "R45-2-cRIO\\global R45_2 shared var lib.lvlib\\R45 Vac cluster 2 Ion Gauge Interlock"(w268) -> ()  [unwired: 1 in, 1 out]
    n175 = shared-variable "R45-2-cRIO\\global R45_2 shared var lib.lvlib\\R45 Vac cluster 4 Ion Gauge Interlock"(w269) -> ()  [unwired: 1 in, 1 out]
    n176 = shared-variable "R45-2-cRIO\\global R45_2 shared var lib.lvlib\\R45 Vac cluster 3 Ion Gauge Interlock"(w270) -> ()  [unwired: 1 in, 1 out]
    n177 = shared-variable ".\\local R45_2 shared var lib.lvlib\\Interlock readback loop error"(w266) -> ()  [unwired: 1 in, 1 out]
  }
  n178 = while {
    tunnel: w2 -> [w299]
    tunnel: w1 -> [w277]
    stop <- FALSE stop-if-true
    # "Error Reporting\nRT error value sets blinking rate USER FPGA LED on cRIO chassis (no error: 0.5 Hz; error: 5 Hz)"
    n179 = xnode "Read/Write Control"("FPGA VI Reference In"=w299) -> ("FPGA VI Reference Out"=w298:refnum<k20>, "error out"=w297:errorcluster, "ExB 1 PS error"=w296:errorcluster, "ExB 2 PS error"=w295:errorcluster, "GFM ps error"=w294:errorcluster, "GFM Hall Probe error"=w293:errorcluster, "HV Readback Loop"=w292:errorcluster, "HV Control Loop error"=w291:errorcluster, "Vacuum Gauge 2 error"=w276:errorcluster, "Vacuum Gauge 3 error"=w275:errorcluster, "Vacuum Gauge 4 error"=w274:errorcluster, "Vac and GV  interlock error"=w287:errorcluster, "Position-Status Sensor error"=w288:errorcluster, "Cup-Aperture Control Loop Error"=w289:errorcluster)  [unwired: 1 in]
    n180 = shared-variable ".\\local R45_2 shared var lib.lvlib\\Interlock readback loop error"() -> (w279:errorcluster)  [unwired: 1 in, 1 out]
    n181 = shared-variable ".\\local R45_2 shared var lib.lvlib\\Vacuum Readback loop error"() -> (w283:errorcluster)  [unwired: 1 in, 1 out]
    n182 = shared-variable ".\\local R45_2 shared var lib.lvlib\\Actuator-Sensor loop error"() -> (w278:errorcluster)  [unwired: 1 in, 1 out]
    n183 = shared-variable ".\\local R45_2 shared var lib.lvlib\\HV readback loop error"() -> (w285:errorcluster)  [unwired: 1 in, 1 out]
    n184 = shared-variable ".\\local R45_2 shared var lib.lvlib\\HV control loop error"() -> (w284:errorcluster)  [unwired: 1 in, 1 out]
    n185 = shared-variable ".\\local R45_2 shared var lib.lvlib\\ExB 1 PS loop error"() -> (w280:errorcluster)  [unwired: 1 in, 1 out]
    n186 = shared-variable ".\\local R45_2 shared var lib.lvlib\\ExB 2 PS loop error"() -> (w281:errorcluster)  [unwired: 1 in, 1 out]
    n187 = shared-variable ".\\local R45_2 shared var lib.lvlib\\GFM loop error"() -> (w282:errorcluster)  [unwired: 1 in, 1 out]
    n188 = Merge Errors(w297, w296, w295, w294, w293, w292, w291, w276, w275, w274, w287, w288, w289) -> (w301:errorcluster)
    n189 = Merge Errors(w277, w278, w279, w280, w281, w282, w283, w284, w285) -> (w272:errorcluster)
    n190 = shared-variable "R45-2-cRIO\\global R45_2 shared var lib.lvlib\\R45-2-FPGA Error"(w301) -> ()  [unwired: 1 in, 1 out]
    n191 = shared-variable "R45-2-cRIO\\global R45_2 shared var lib.lvlib\\R45-2-RT Error"(w272) -> ()  [unwired: 1 in, 1 out]
    n192 = Unbundle By Name(w301) -> ("status"=w300:bool)
    n193 = case shown="Error" w272 {
      tunnel: 0 -> [w304 w312]
      frame No Error {
        n194 = flat-sequence {
          tunnel: w304 -> [w305]
          tunnel: [w305] -> w302
          tunnel: [w307] -> w303
          tunnel: w302 -> [w307]
          tunnel: w303 -> [w309]
          frame #0 {
            n195 = call <vilib>:"RT LEDs.vi"("State"=3, "LED Num"=w305) -> ()  [unwired: 4 in, 2 out]
          }
          frame #1 {
            n196 = call "Wait Until Next Multiple7"("Count(mSec)"=u16 1000) -> ()  [unwired: 1 out]
          }
          frame #2 {
            n197 = call <vilib>:"RT LEDs.vi"("State"=3, "LED Num"=w309) -> ()  [unwired: 4 in, 2 out]
          }
          frame #3 {
            n198 = call "Wait Until Next Multiple10"("Count(mSec)"=u16 1000) -> ()  [unwired: 1 out]
          }
        }
      }
      frame Error {
        n199 = flat-sequence {
          tunnel: [w315] -> w314
          tunnel: w312 -> [w315]
          tunnel: w314 -> [w317]
          tunnel: [w317] -> w313
          tunnel: w313 -> [w319]
          frame #0 {
            n200 = call <vilib>:"RT LEDs.vi"("State"=3, "LED Num"=w315) -> ()  [unwired: 4 in, 2 out]
          }
          frame #1 {
            n201 = call "Wait Until Next Multiple11"("Count(mSec)"=u16 100) -> ()  [unwired: 1 out]
          }
          frame #2 {
            n202 = call <vilib>:"RT LEDs.vi"("State"=3, "LED Num"=w319) -> ()  [unwired: 4 in, 2 out]
          }
          frame #3 {
            n203 = call "Wait Until Next Multiple12"("Count(mSec)"=u16 100) -> ()  [unwired: 1 out]
          }
        }
      }
    }
    n204 = Merge Errors(w272, w301) -> (→"Error Reporter":errorcluster)
    n205 = xnode "Read/Write Control"("FPGA VI Reference In"=w298, "RT error"=w300) -> ()  [unwired: 1 in, 2 out]
  }
